vi "Write Payload.vi"(10 "Payload":string, 11 "GDSII.DataType.Long in":refnum<class "GDSII.DataType.Long.lvclass">) -> (3 "GDSII.DataType.Long out":refnum<class "GDSII.DataType.Long.lvclass">)   [LabVIEW 2019, in "GDSII.DataType.Long.lvclass"]
uses:
  GDSII.DataType.Long.lvclass
  GDSII.DataType.Long.lvclass/GDSII.DataType.Long.ctl
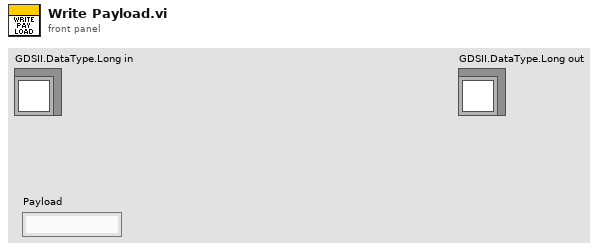
[diagram p1: front panel]
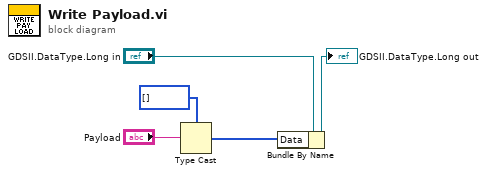
[diagram p0: block diagram]
diagram:
  n1 = Type Cast(type=i32[] [] ("Data"), x="Payload") -> (*(type *) &x=w1:i32[])
  n2 = Bundle By Name(cluster="GDSII.DataType.Long in", "Data"=w1) -> (→"GDSII.DataType.Long out":refnum<class "GDSII.DataType.Long.lvclass">)
